vi "problem 1.vi"() -> ()   [LabVIEW 2015]
panel:
  in  "stop":bool
  out "String":string
  out "output":dbl
  in  "operation":dbl
  in  "number 2":dbl
  in  "number 1":dbl
  # "select operation\n 1.Addition 2.subtraction 3.multiplication 4.division\n5.Square 6.squareroot"
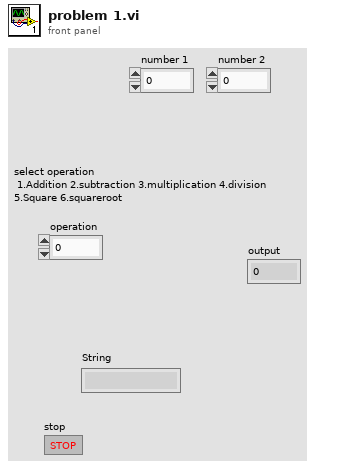
[diagram p1: front panel]
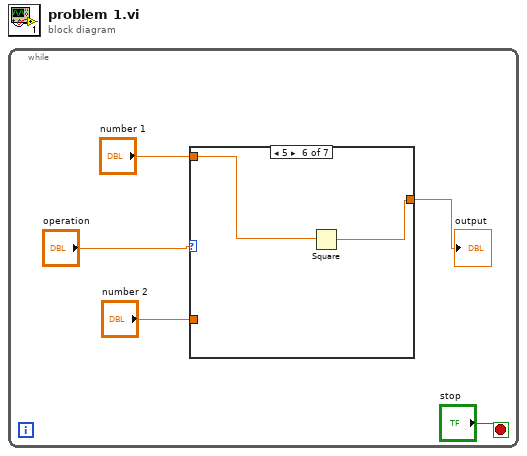
[diagram p0: block diagram]
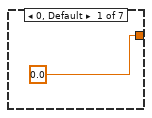
[diagram p2: hidden frame]
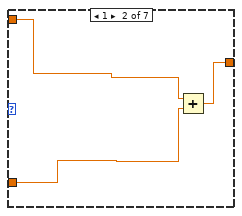
[diagram p3: hidden frame]
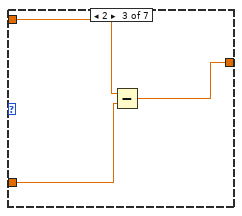
[diagram p4: hidden frame]
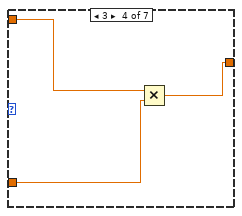
[diagram p5: hidden frame]
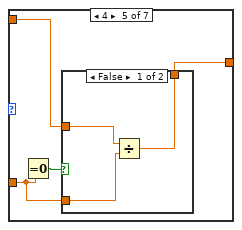
[diagram p6: hidden frame]
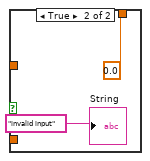
[diagram p7: hidden frame]
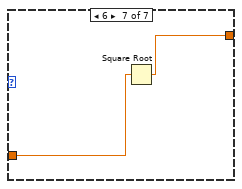
[diagram p8: hidden frame]
diagram:
  n1 = while {
    stop <- "stop" stop-if-true
    n2 = case shown="5" "operation" {
      tunnel: [0.0 ("operation 2") w9 w10 w13 w18 w25 w28] -> w4
      tunnel: "number 1" -> [_ w8 w12 w15 w17 w26 _]
      tunnel: "number 2" -> [_ w7 w11 w14 w19 _ w27]
      frame 0, Default {
      }
      frame 1 {
        n3 = Add(x=w8, y=w7) -> (x+y=w9:dbl)
      }
      frame 2 {
        n4 = Subtract(x=w12, y=w11) -> (x-y=w10:dbl)
      }
      frame 3 {
        n5 = Multiply(x=w15, y=w14) -> (x*y=w13:dbl)
      }
      frame 4 {
        n6 = Equal To 0?(x=w19) -> (x = 0?=w16:bool)
        n7 = case shown="False" w16 {
          tunnel: [w20 0.0 ("Numeric")] -> w18
          tunnel: w19 -> [w21 _]
          tunnel: w17 -> [w22 _]
          frame False {
            n8 = Divide(x=w22, y=w21) -> (x/y=w20:dbl)
          }
          frame True {
            "String" <- "invalid input"
          }
        }
      }
      frame 5 {
        n9 = Square(x=w26) -> (x^2=w25:dbl)
      }
      frame 6 {
        n10 = Square Root(x=w27) -> (sqrt(x)=w28:dbl)
      }
    }
    "output" <- w4
  }
